vi "Display Values (SubVI).vi"(0 "Channels List":refnum<k21>, 1 "All Names":string[](array[string]), 2 "# PT":i32, 3 "# MFC":i32, 4 "# RH (T) Probes":i32, 5 "error In":errorcluster, 6 "# TC (NI)":i32, 7 "# RH Probes":i32, 8 "PT Units In":string[](array[string])) -> (9 "NI TC Names":string[](array[string]), 10 "RH (T) Units":i32[](array[numeric]), 11 "PT Units Out":string[](array[string]), 12 "NI TC Units":i32[](array[numeric]), 13 "RH (T) Names":string[](array[string]), 14 "RH Names":string[](array[string]), 15 "MFC Names":string[](array[string]), 16 "PT Names":string[](array[string]), 17 "RH Units":string[](array[string]), 18 "MFC Units":string[](array[string]), 19 "error out":errorcluster)   [LabVIEW 2011]
uses:
  <vilib>/Utility/error.llb/DialogType.ctl
  Program Files (x86)/National Instruments/LabVIEW 2011/resource/objmgr/daqmx.rc
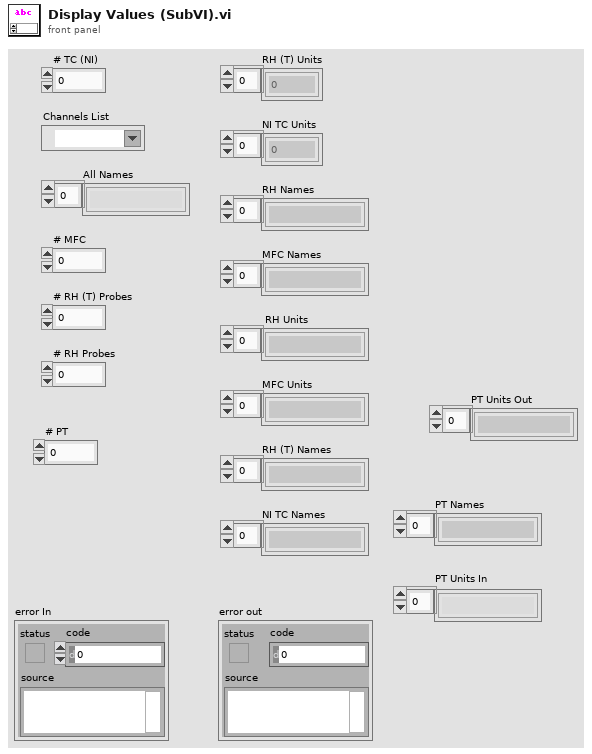
[diagram p1: front panel]
types:
  T1 = typedef "DialogType.ctl" = u16
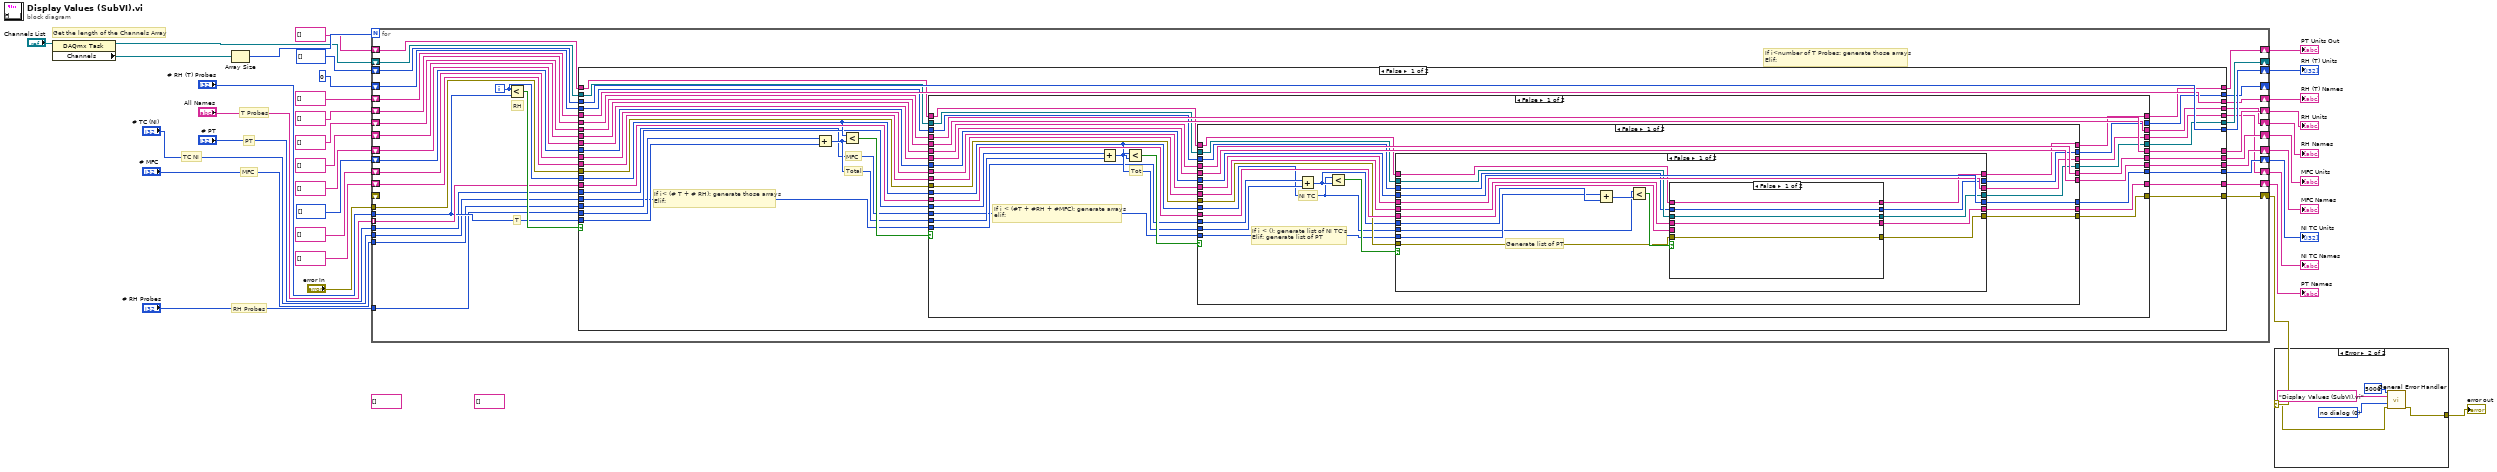
[diagram p0: block diagram]
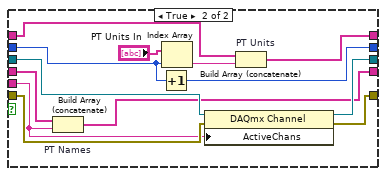
[diagram p3: hidden frame]
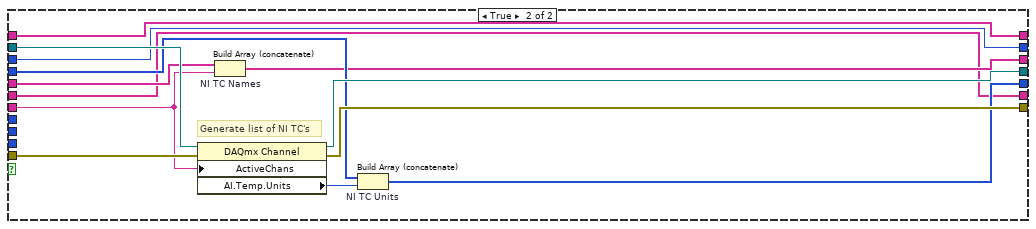
[diagram p4: hidden frame]
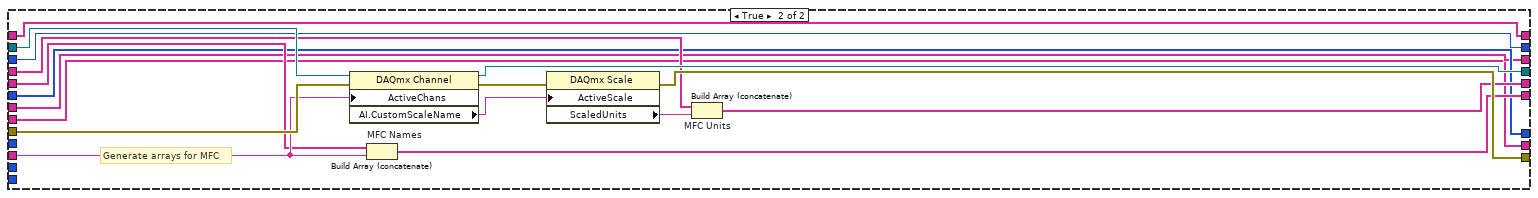
[diagram p5: hidden frame]
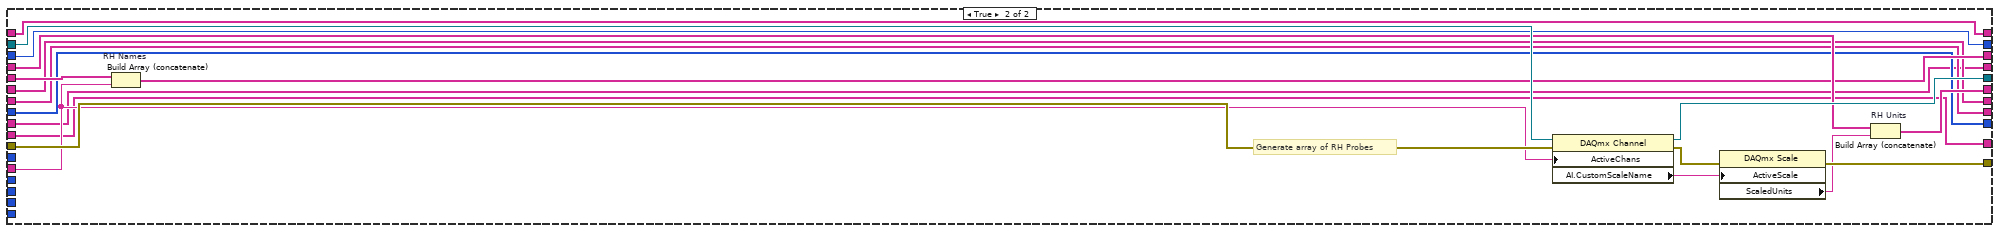
[diagram p6: hidden frame]
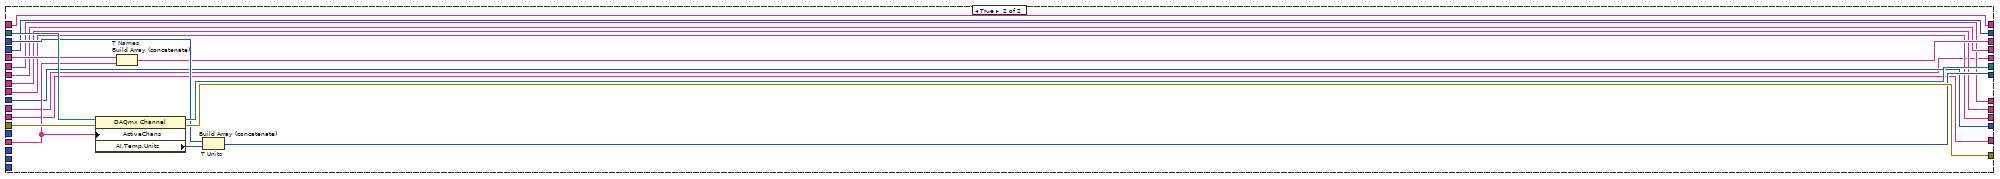
[diagram p7: hidden frame]
diagram:
  (unwired) string[] []
  (unwired) string[] []
  # "PT"
  # "TC NI"
  # "MFC"
  # "RH Probes"
  # "T Probes"
  # "Get the length of the Channels Array"
  n1 = property class="DAQmx Task"(reference="Channels List") -> (reference out=w27:refnum<k21>, "Channels"=w32:refnum<k21>[])  [unwired: 1 in, 1 out]
  n2 = Array Size(array=w32) -> (size(s)=w33:i32)
  n3 = for {
    N: w33 -> [_]
    tunnel: "# RH (T) Probes" -> [w57]
    tunnel: "# RH Probes" -> [w56]
    tunnel: "# MFC" -> [w51]
    tunnel: "# TC (NI)" -> [w46]
    tunnel: "# PT" -> [w41]
    tunnel: "error In" -> [w67]
    shift-right: [w66] -> w2
    shift-left: _ -> [_]
    shift-right: [w65] -> _
    shift-left: w27 -> [w64]
    tunnel: "All Names" -> [w63] mode=indexing
    shift-right: [w62] -> w6
    shift-left: i32[] [] -> [w61]
    shift-right: [w60] -> w9
    shift-left: string[] [] -> [w59]
    shift-right: [w55] -> w5
    shift-left: string[] [] -> [w54]
    shift-right: [w53] -> w12
    shift-left: string[] [] -> [w52]
    shift-right: [w50] -> w4
    shift-left: string[] [] -> [w49]
    shift-right: [w48] -> w11
    shift-left: string[] [] -> [w47]
    shift-right: [w45] -> w3
    shift-left: i32[] [] -> [w44]
    shift-right: [w43] -> w10
    shift-left: string[] [] -> [w42]
    shift-right: [w40] -> _
    shift-left: 0 -> [w39]
    shift-right: [w38] -> w8
    shift-left: string[] [] -> [w37]
    shift-right: [w36] -> w7
    shift-left: string[] [] -> [w35]
    i -> [w58]
    # "T"
    # "RH"
    # "If i<number of T Probes: generate those arrays\nElif:"
    n4 = Less?(x=w58, y=w57) -> (x < y?=w68:bool)
    n5 = case shown="False" w68 {
      tunnel: w67 -> [w94 w256]
      tunnel: [w93 w255] -> w66
      tunnel: [w95 w254] -> w65
      tunnel: w64 -> [w96 w253]
      tunnel: w63 -> [w92 w247]
      tunnel: [w101 w252] -> w62
      tunnel: w61 -> [w101 w251]
      tunnel: [w100 w249] -> w60
      tunnel: w59 -> [w100 w248]
      tunnel: w58 -> [w87 _]
      tunnel: w57 -> [w98 _]
      tunnel: w56 -> [w97 _]
      tunnel: [w91 w245] -> w55
      tunnel: w54 -> [w90 w245]
      tunnel: [w89 w246] -> w53
      tunnel: w52 -> [w88 w246]
      tunnel: w51 -> [w85 _]
      tunnel: [w84 w244] -> w50
      tunnel: w49 -> [w83 w244]
      tunnel: [w82 w243] -> w48
      tunnel: w47 -> [w81 w243]
      tunnel: w46 -> [w80 _]
      tunnel: [w79 w242] -> w45
      tunnel: w44 -> [w78 w242]
      tunnel: [w77 w241] -> w43
      tunnel: w42 -> [w76 w241]
      tunnel: w41 -> [w75 _]
      tunnel: [w74 w240] -> w40
      tunnel: w39 -> [w73 w240]
      tunnel: [w72 w239] -> w38
      tunnel: w37 -> [w71 w239]
      tunnel: [w70 w238] -> w36
      tunnel: w35 -> [w69 w238]
      frame False {
        # "MFC"
        # "Total"
        # "If i< (# T + # RH): generate those arrays\nElif:"
        n6 = Add(x=w97, y=w98) -> (x+y=w86:i32)
        n7 = Less?(x=w87, y=w86) -> (x < y?=w99:bool)
        n8 = case shown="False" w99 {
          tunnel: w96 -> [w124 w237]
          tunnel: [w123 w236] -> w95
          tunnel: w94 -> [w122 w235]
          tunnel: [w121 w233] -> w93
          tunnel: w92 -> [w120 w226]
          tunnel: [w129 w230] -> w91
          tunnel: w90 -> [w129 w229]
          tunnel: [w128 w228] -> w89
          tunnel: w88 -> [w128 w227]
          tunnel: w87 -> [w113 _]
          tunnel: w86 -> [w126 _]
          tunnel: w85 -> [w125 _]
          tunnel: [w119 w224] -> w84
          tunnel: w83 -> [w118 w224]
          tunnel: [w117 w225] -> w82
          tunnel: w81 -> [w116 w225]
          tunnel: w80 -> [w114 _]
          tunnel: [w112 w223] -> w79
          tunnel: w78 -> [w111 w223]
          tunnel: [w110 w222] -> w77
          tunnel: w76 -> [w109 w222]
          tunnel: w75 -> [w108 _]
          tunnel: [w107 w221] -> w74
          tunnel: w73 -> [w106 w221]
          tunnel: [w105 w220] -> w72
          tunnel: w71 -> [w104 w220]
          tunnel: [w103 w219] -> w70
          tunnel: w69 -> [w102 w219]
          frame False {
            # "Tot"
            # "If i < (#T + #RH + #MFC): generate arrays\nelif:"
            n9 = Add(x=w125, y=w126) -> (x+y=w115:i32)
            n10 = Less?(x=w113, y=w115) -> (x < y?=w127:bool)
            n11 = case shown="False" w127 {
              tunnel: w124 -> [w145 w218]
              tunnel: [w143 w217] -> w123
              tunnel: w122 -> [w146 w216]
              tunnel: [w144 w214] -> w121
              tunnel: w120 -> [w147 w209]
              tunnel: [w151 w211] -> w119
              tunnel: w118 -> [w151 w210]
              tunnel: [w152 w208] -> w117
              tunnel: w116 -> [w152 w207]
              tunnel: w115 -> [w149 _]
              tunnel: w114 -> [w148 _]
              tunnel: w113 -> [w136 _]
              tunnel: [w142 w206] -> w112
              tunnel: w111 -> [w141 w206]
              tunnel: [w140 w205] -> w110
              tunnel: w109 -> [w139 w205]
              tunnel: w108 -> [w137 _]
              tunnel: [w135 w204] -> w107
              tunnel: w106 -> [w134 w204]
              tunnel: [w133 w203] -> w105
              tunnel: w104 -> [w132 w203]
              tunnel: [w131 w202] -> w103
              tunnel: w102 -> [w130 w202]
              frame False {
                # "NI TC"
                # "If i < (): generate list of NI TC's\nElif: generate list of PT"
                n12 = Add(x=w148, y=w149) -> (x+y=w138:i32)
                n13 = Less?(x=w136, y=w138) -> (x < y?=w150:bool)
                n14 = case shown="False" w150 {
                  tunnel: w147 -> [w162 w194]
                  tunnel: w146 -> [w163 w199]
                  tunnel: w145 -> [w161 w201]
                  tunnel: [w159 w198] -> w144
                  tunnel: [w160 w200] -> w143
                  tunnel: [w170 w196] -> w142
                  tunnel: w141 -> [w170 w195]
                  tunnel: [w169 w193] -> w140
                  tunnel: w139 -> [w169 w192]
                  tunnel: w138 -> [w168 _]
                  tunnel: w137 -> [w165 _]
                  tunnel: w136 -> [w164 _]
                  tunnel: [w158 w191] -> w135
                  tunnel: w134 -> [w157 w191]
                  tunnel: [w156 w190] -> w133
                  tunnel: w132 -> [w155 w190]
                  tunnel: [w154 w189] -> w131
                  tunnel: w130 -> [w153 w189]
                  frame False {
                    # "Generate list of PT"
                    n15 = Add(x=w165, y=w168) -> (x+y=w167:i32)
                    n16 = Less?(x=w164, y=w167) -> (x < y?=w166:bool)
                    n17 = case shown="False" w166 {
                      tunnel: w163 -> [w175 w187]
                      tunnel: w162 -> [_ w183]
                      tunnel: w161 -> [w174 w186]
                      tunnel: [w174 w185] -> w160
                      tunnel: [w175 w184] -> w159
                      tunnel: [w173 w188] -> w158
                      tunnel: w157 -> [w173 w179]
                      tunnel: [w171 w182] -> w156
                      tunnel: w155 -> [w171 w181]
                      tunnel: [w172 w177] -> w154
                      tunnel: w153 -> [w172 w176]
                      frame False {
                      }
                      frame True {
                        n18 = Build Array (concatenate) "PT Names"(w181, w183) -> (w182:string[])
                        n19 = Increment(x=w179) -> (x+1=w188:i32)
                        n20 = Index Array(array="PT Units In", index=w179) -> (element=w178:string)
                        n21 = property class="DAQmx Channel"(reference=w186, error in=w187, "ActiveChans"=w183) -> (reference out=w185:refnum<k21>, error out=w184:errorcluster)
                        n22 = Build Array (concatenate) "PT Units"(w176, w178) -> (w177:string[])
                      }
                    }
                  }
                  frame True {
                    # "Generate list of NI TC's"
                    n23 = property class="DAQmx Channel"(reference=w201, error in=w199, "ActiveChans"=w194) -> (reference out=w200:refnum<k21>, error out=w198:errorcluster, "AI.Temp.Units"=w197:i32)
                    n24 = Build Array (concatenate) "NI TC Names"(w192, w194) -> (w193:string[])
                    n25 = Build Array (concatenate) "NI TC Units"(w195, w197) -> (w196:i32[])
                  }
                }
              }
              frame True {
                # "Generate arrays for MFC"
                n26 = property class="DAQmx Channel"(reference=w218, error in=w216, "ActiveChans"=w209) -> (reference out=w217:refnum<k21>, error out=w215:errorcluster, "AI.CustomScaleName"=w213:tag)
                n27 = Build Array (concatenate) "MFC Names"(w207, w209) -> (w208:string[])
                n28 = property class="DAQmx Scale"(error in=w215, "ActiveScale"=w213) -> (error out=w214:errorcluster, "ScaledUnits"=w212:string)  [unwired: 1 in, 1 out]
                n29 = Build Array (concatenate) "MFC Units"(w210, w212) -> (w211:string[])
              }
            }
          }
          frame True {
            # "Generate array of RH Probes"
            n30 = Build Array (concatenate) "RH Names"(w227, w226) -> (w228:string[])
            n31 = property class="DAQmx Channel"(reference=w237, error in=w235, "ActiveChans"=w226) -> (reference out=w236:refnum<k21>, error out=w234:errorcluster, "AI.CustomScaleName"=w232:tag)
            n32 = property class="DAQmx Scale"(error in=w234, "ActiveScale"=w232) -> (error out=w233:errorcluster, "ScaledUnits"=w231:string)  [unwired: 1 in, 1 out]
            n33 = Build Array (concatenate) "RH Units"(w229, w231) -> (w230:string[])
          }
        }
      }
      frame True {
        n34 = property class="DAQmx Channel"(reference=w253, error in=w256, "ActiveChans"=w247) -> (reference out=w254:refnum<k21>, error out=w255:errorcluster, "AI.Temp.Units"=w250:i32)
        n35 = Build Array (concatenate) "T Names"(w248, w247) -> (w249:string[])
        n36 = Build Array (concatenate) "T Units"(w251, w250) -> (w252:i32[])
      }
    }
  }
  "MFC Units" <- w4
  "MFC Names" <- w11
  "RH Units" <- w5
  "RH Names" <- w12
  "NI TC Units" <- w3
  "RH (T) Units" <- w6
  "NI TC Names" <- w10
  "RH (T) Names" <- w9
  "PT Units Out" <- w7
  "PT Names" <- w8
  n37 = case shown="Error" w2 {
    selector: w2 -> [w257 w261]
    tunnel: [w257 w262] -> w1
    frame No Error {
    }
    frame Error {
      w258 = T1 0 items=["no dialog", "OK message", "continue or stop message", "OK message + warnings", "continue/stop + warnings"] ("type of dialog (OK msg:1)")
      n38 = call <vilib>:"General Error Handler.vi"("[error code] (0)"=5006, "[error source] (\" \")"="Display Values (SubVI).vi" ("[error source] (\" \")"), "type of dialog (OK msg:1)"=w258, "error in (no error)"=w261) -> ("error out"=w262:errorcluster)  [unwired: 7 in, 4 out]
    }
  }
  "error out" <- w1
